vi "semester_1_project_server.vi"   [LabVIEW 2024]
uses:
  semester_1_project_global.vi
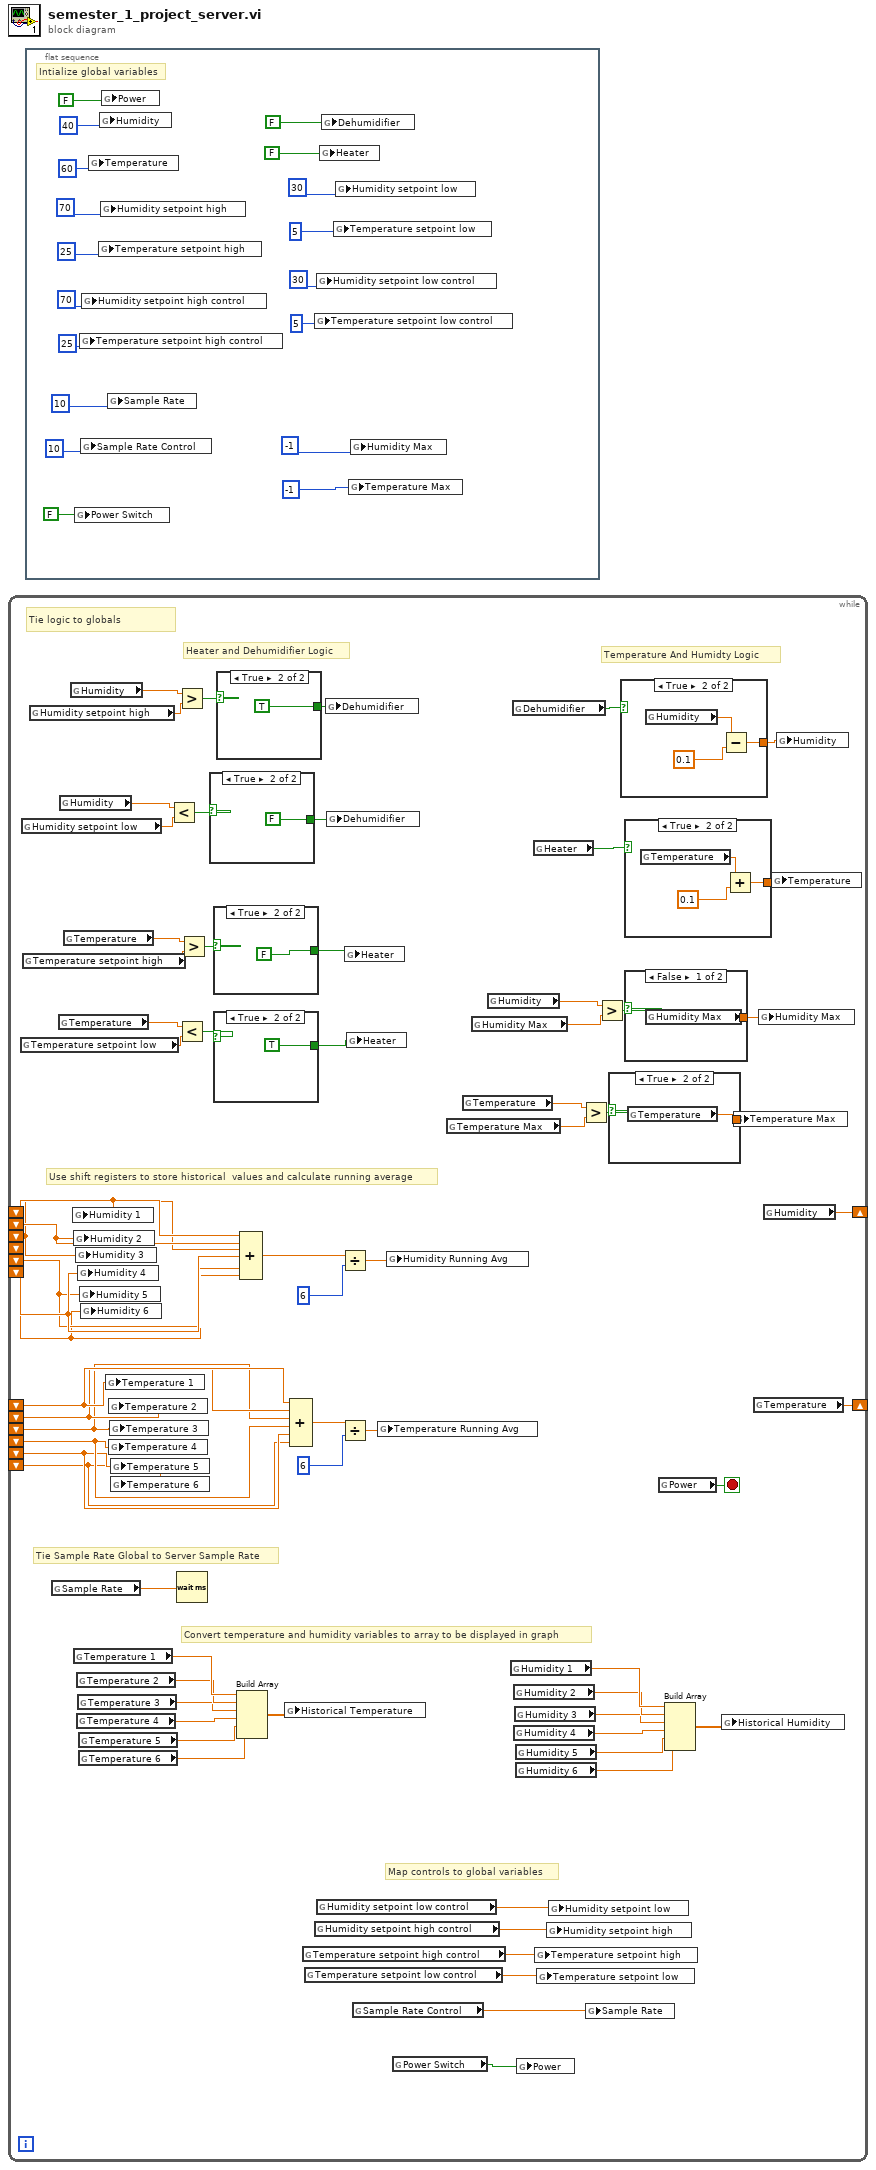
[diagram p0: block diagram]
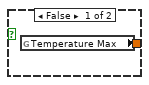
[diagram p2: hidden frame]
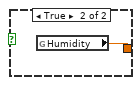
[diagram p3: hidden frame]
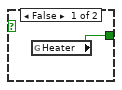
[diagram p4: hidden frame]
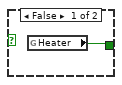
[diagram p5: hidden frame]
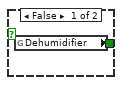
[diagram p6: hidden frame]
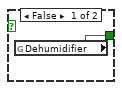
[diagram p7: hidden frame]
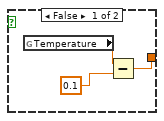
[diagram p8: hidden frame]
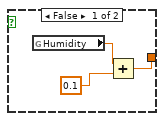
[diagram p9: hidden frame]
diagram:
  n1 = while {
    shift-right: [w48] -> _
    shift-left: _ -> [w46]
    shift-left: _ -> [w45]
    shift-left: _ -> [w44]
    shift-left: _ -> [w43]
    shift-left: _ -> [w42]
    shift-left: _ -> [w41]
    shift-right: [w47] -> _
    shift-left: _ -> [w35]
    shift-left: _ -> [w34]
    shift-left: _ -> [w33]
    shift-left: _ -> [w32]
    shift-left: _ -> [w31]
    shift-left: _ -> [w30]
    stop <- w69 stop-if-true
    # "Heater and Dehumidifier Logic"
    # "Temperature And Humidty Logic"
    # "Use shift registers to store historical  values and calculate running average"
    # "Tie Sample Rate Global to Server Sample Rate"
    # "Map controls to global variables"
    # "Convert temperature and humidity variables to array to be displayed in graph"
    # "Tie logic to globals"
    n2 = global read "semester_1_project_global.vi" "Temperature setpoint low"() -> (w51:dbl)
    n3 = global read "semester_1_project_global.vi" "Humidity setpoint low"() -> (w59:dbl)
    n4 = global read "semester_1_project_global.vi" "Temperature setpoint high"() -> (w55:dbl)
    n5 = global read "semester_1_project_global.vi" "Humidity setpoint high"() -> (w67:dbl)
    n6 = global read "semester_1_project_global.vi" "Sample Rate"() -> (w70:dbl)
    n7 = global read "semester_1_project_global.vi" "Temperature"() -> (w52:dbl)
    n8 = global read "semester_1_project_global.vi" "Humidity"() -> (w60:dbl)
    n9 = global read "semester_1_project_global.vi" "Temperature"() -> (w56:dbl)
    n10 = global read "semester_1_project_global.vi" "Humidity"() -> (w68:dbl)
    n11 = global write "semester_1_project_global.vi" "Humidity 1"(w46) -> ()
    n12 = global write "semester_1_project_global.vi" "Humidity 2"(w45) -> ()
    n13 = global read "semester_1_project_global.vi" "Temperature 1"() -> (w20:dbl)
    n14 = global write "semester_1_project_global.vi" "Humidity 3"(w44) -> ()
    n15 = global read "semester_1_project_global.vi" "Temperature 2"() -> (w19:dbl)
    n16 = global read "semester_1_project_global.vi" "Temperature 4"() -> (w17:dbl)
    n17 = global write "semester_1_project_global.vi" "Humidity 4"(w43) -> ()
    n18 = global read "semester_1_project_global.vi" "Temperature 3"() -> (w18:dbl)
    n19 = global read "semester_1_project_global.vi" "Temperature 5"() -> (w16:dbl)
    n20 = global read "semester_1_project_global.vi" "Temperature 6"() -> (w14:dbl)
    n21 = global write "semester_1_project_global.vi" "Humidity 5"(w42) -> ()
    n22 = global write "semester_1_project_global.vi" "Humidity 6"(w41) -> ()
    n23 = global write "semester_1_project_global.vi" "Temperature 1"(w35) -> ()
    n24 = global write "semester_1_project_global.vi" "Temperature 2"(w34) -> ()
    n25 = global write "semester_1_project_global.vi" "Temperature 4"(w32) -> ()
    n26 = global write "semester_1_project_global.vi" "Temperature 3"(w33) -> ()
    n27 = global write "semester_1_project_global.vi" "Temperature 5"(w31) -> ()
    n28 = global write "semester_1_project_global.vi" "Temperature 6"(w30) -> ()
    n29 = Less?(x=w60, y=w59) -> (x < y?=w58:bool)
    n30 = Greater?(x=w68, y=w67) -> (0:w62:bool)
    n31 = Less?(x=w52, y=w51) -> (x < y?=w50:bool)
    n32 = Wait (ms)(milliseconds to wait=w70) -> ()  [unwired: 1 out]
    n33 = Greater?(x=w56, y=w55) -> (0:w54:bool)
    n34 = case shown="True" w58 {
      tunnel: [w79 FALSE] -> w57
      frame False {
        n35 = global read "semester_1_project_global.vi" "Dehumidifier"() -> (w79:bool)
      }
      frame True {
      }
    }
    n36 = case shown="True" w54 {
      tunnel: [w77 FALSE] -> w53
      frame False {
        n37 = global read "semester_1_project_global.vi" "Heater"() -> (w77:bool)
      }
      frame True {
      }
    }
    n38 = case shown="True" w50 {
      tunnel: [w75 TRUE] -> w49
      frame False {
        n39 = global read "semester_1_project_global.vi" "Heater"() -> (w75:bool)
      }
      frame True {
      }
    }
    n40 = case shown="True" w62 {
      tunnel: [w81 TRUE] -> w61
      frame False {
        n41 = global read "semester_1_project_global.vi" "Dehumidifier"() -> (w81:bool)
      }
      frame True {
      }
    }
    n42 = Build Array(w20, w19, w18, w17, w16, w14) -> (w15:dbl[])
    n43 = Compound Arithmetic op=ADD(w46, w45, w44, w43, w42, w41) -> (w40:dbl)
    n44 = global write "semester_1_project_global.vi" "Historical Temperature"(w15) -> ()
    n45 = Compound Arithmetic op=ADD(w35, w34, w33, w32, w31, w30) -> (w29:dbl)
    n46 = global read "semester_1_project_global.vi" "Temperature setpoint high control"() -> (w3:dbl)
    n47 = global read "semester_1_project_global.vi" "Temperature setpoint low control"() -> (w2:dbl)
    n48 = global read "semester_1_project_global.vi" "Humidity setpoint high control"() -> (w4:dbl)
    n49 = global read "semester_1_project_global.vi" "Humidity setpoint low control"() -> (w5:dbl)
    n50 = global write "semester_1_project_global.vi" "Dehumidifier"(w61) -> ()
    n51 = global write "semester_1_project_global.vi" "Dehumidifier"(w57) -> ()
    n52 = Divide(x=w40, y=6) -> (x/y=w38:dbl)
    n53 = Divide(x=w29, y=6) -> (x/y=w36:dbl)
    n54 = global write "semester_1_project_global.vi" "Heater"(w53) -> ()
    n55 = global write "semester_1_project_global.vi" "Heater"(w49) -> ()
    n56 = global read "semester_1_project_global.vi" "Sample Rate Control"() -> (w1:dbl)
    n57 = global write "semester_1_project_global.vi" "Temperature Running Avg"(w36) -> ()
    n58 = global write "semester_1_project_global.vi" "Humidity Running Avg"(w38) -> ()
    n59 = global read "semester_1_project_global.vi" "Power Switch"() -> (w6:bool)
    n60 = global read "semester_1_project_global.vi" "Temperature Max"() -> (w23:dbl)
    n61 = global read "semester_1_project_global.vi" "Temperature"() -> (w24:dbl)
    n62 = global read "semester_1_project_global.vi" "Humidity Max"() -> (w27:dbl)
    n63 = global read "semester_1_project_global.vi" "Humidity"() -> (w28:dbl)
    n64 = global read "semester_1_project_global.vi" "Humidity 1"() -> (w13:dbl)
    n65 = global read "semester_1_project_global.vi" "Dehumidifier"() -> (w65:bool)
    n66 = global read "semester_1_project_global.vi" "Humidity 2"() -> (w12:dbl)
    n67 = global read "semester_1_project_global.vi" "Humidity 4"() -> (w10:dbl)
    n68 = global read "semester_1_project_global.vi" "Humidity 3"() -> (w11:dbl)
    n69 = global read "semester_1_project_global.vi" "Humidity 5"() -> (w9:dbl)
    n70 = global read "semester_1_project_global.vi" "Humidity 6"() -> (w7:dbl)
    n71 = global write "semester_1_project_global.vi" "Power"(w6) -> ()
    n72 = global read "semester_1_project_global.vi" "Heater"() -> (w63:bool)
    n73 = global write "semester_1_project_global.vi" "Temperature setpoint high"(w3) -> ()
    n74 = global write "semester_1_project_global.vi" "Temperature setpoint low"(w2) -> ()
    n75 = global write "semester_1_project_global.vi" "Humidity setpoint high"(w4) -> ()
    n76 = global write "semester_1_project_global.vi" "Humidity setpoint low"(w5) -> ()
    n77 = Greater?(x=w24, y=w23) -> (0:w22:bool)
    n78 = global write "semester_1_project_global.vi" "Sample Rate"(w1) -> ()
    n79 = Greater?(x=w28, y=w27) -> (0:w26:bool)
    n80 = case shown="True" w22 {
      tunnel: [w71 w72] -> w21
      frame False {
        n81 = global read "semester_1_project_global.vi" "Temperature Max"() -> (w71:dbl)
      }
      frame True {
        n82 = global read "semester_1_project_global.vi" "Temperature"() -> (w72:dbl)
      }
    }
    n83 = case shown="True" w65 {
      tunnel: [w89 w92] -> w66
      frame False {
        n84 = global read "semester_1_project_global.vi" "Humidity"() -> (w90:dbl)
        n85 = Add(x=w90, y=0.1) -> (x+y=w89:dbl)
      }
      frame True {
        n86 = global read "semester_1_project_global.vi" "Humidity"() -> (w94:dbl)
        n87 = Subtract(x=w94, y=0.1) -> (x-y=w92:dbl)
      }
    }
    n88 = case shown="True" w63 {
      tunnel: [w83 w86] -> w64
      frame False {
        n89 = global read "semester_1_project_global.vi" "Temperature"() -> (w84:dbl)
        n90 = Subtract(x=w84, y=0.1) -> (x-y=w83:dbl)
      }
      frame True {
        n91 = global read "semester_1_project_global.vi" "Temperature"() -> (w88:dbl)
        n92 = Add(x=w88, y=0.1) -> (x+y=w86:dbl)
      }
    }
    n93 = case shown="False" w26 {
      tunnel: [w73 w74] -> w25
      frame False {
        n94 = global read "semester_1_project_global.vi" "Humidity Max"() -> (w73:dbl)
      }
      frame True {
        n95 = global read "semester_1_project_global.vi" "Humidity"() -> (w74:dbl)
      }
    }
    n96 = global read "semester_1_project_global.vi" "Power"() -> (w69:bool)
    n97 = Build Array(w13, w12, w11, w10, w9, w7) -> (w8:dbl[])
    n98 = global write "semester_1_project_global.vi" "Historical Humidity"(w8) -> ()
    n99 = global write "semester_1_project_global.vi" "Temperature Max"(w21) -> ()
    n100 = global read "semester_1_project_global.vi" "Temperature"() -> (w47:dbl)
    n101 = global write "semester_1_project_global.vi" "Humidity Max"(w25) -> ()
    n102 = global read "semester_1_project_global.vi" "Humidity"() -> (w48:dbl)
    n103 = global write "semester_1_project_global.vi" "Temperature"(w64) -> ()
    n104 = global write "semester_1_project_global.vi" "Humidity"(w66) -> ()
  }
  n105 = flat-sequence {
    frame #0 {
      # "Intialize global variables"
      n106 = global write "semester_1_project_global.vi" "Power Switch"(FALSE) -> ()
      n107 = global write "semester_1_project_global.vi" "Temperature setpoint high control"(25) -> ()
      n108 = global write "semester_1_project_global.vi" "Sample Rate Control"(10) -> ()
      n109 = global write "semester_1_project_global.vi" "Humidity setpoint high control"(70) -> ()
      n110 = global write "semester_1_project_global.vi" "Temperature"(60) -> ()
      n111 = global write "semester_1_project_global.vi" "Temperature setpoint high"(25) -> ()
      n112 = global write "semester_1_project_global.vi" "Humidity"(40) -> ()
      n113 = global write "semester_1_project_global.vi" "Humidity setpoint high"(70) -> ()
      n114 = global write "semester_1_project_global.vi" "Power"(FALSE) -> ()
      n115 = global write "semester_1_project_global.vi" "Sample Rate"(10) -> ()
      n116 = global write "semester_1_project_global.vi" "Temperature setpoint low control"(5) -> ()
      n117 = global write "semester_1_project_global.vi" "Humidity setpoint low control"(30) -> ()
      n118 = global write "semester_1_project_global.vi" "Heater"(FALSE) -> ()
      n119 = global write "semester_1_project_global.vi" "Dehumidifier"(FALSE) -> ()
      n120 = global write "semester_1_project_global.vi" "Temperature setpoint low"(5) -> ()
      n121 = global write "semester_1_project_global.vi" "Humidity setpoint low"(30) -> ()
      n122 = global write "semester_1_project_global.vi" "Temperature Max"(-1) -> ()
      n123 = global write "semester_1_project_global.vi" "Humidity Max"(-1) -> ()
    }
  }
